vi "folder_to_string_log_record.vi"(8 "error in":errorcluster, 11 "File Path":path) -> (0 "str_fileerrror":string, 1 "str_fileerased":string, 2 "str_filecopyed":string, 3 "str_foldercreat":string, 4 "str_filenotequal":string)   [LabVIEW 2026]
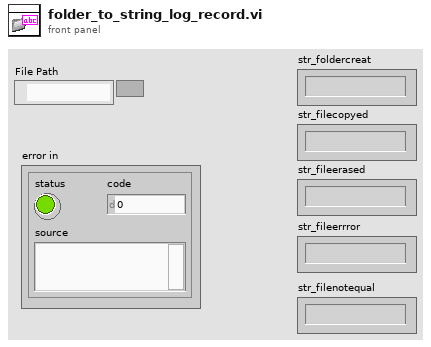
[diagram p1: front panel]
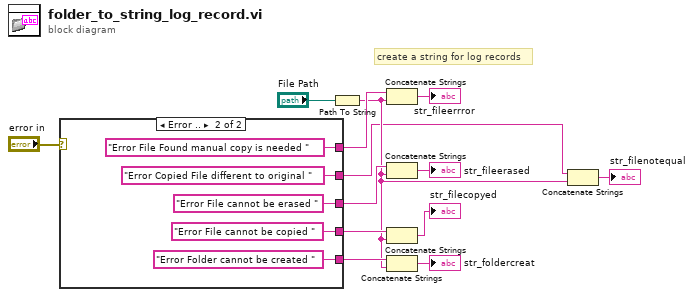
[diagram p0: block diagram]
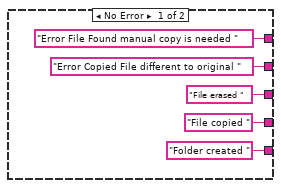
[diagram p2: hidden frame]
diagram:
  # "create a string for log records"
  n1 = case shown="Error .." "error in" {
    tunnel: ["Folder created " "Error Folder cannot be created "] -> w12
    tunnel: ["File copied " "Error File cannot be copied "] -> w10
    tunnel: ["File erased " "Error File cannot be erased "] -> w9
    tunnel: ["Error File Found manual copy is needed " "Error File Found manual copy is needed "] -> w6
    tunnel: ["Error Copied File different to original " "Error Copied File different to original "] -> w2
    frame No Error {
    }
    frame Error {
    }
  }
  n2 = Path To String(path="File Path") -> (string=w3:string)
  n3 = Concatenate Strings(w6, w3) -> (→"str_fileerrror":string)
  n4 = Concatenate Strings(w9, w3) -> (→"str_fileerased":string)
  n5 = Concatenate Strings(w10, w3) -> (→"str_filecopyed":string)
  n6 = Concatenate Strings(w12, w3) -> (→"str_foldercreat":string)
  n7 = Concatenate Strings(w2, w3) -> (→"str_filenotequal":string)
